vi "Process.vi"(8 "error in":errorcluster, 11 "XYStage":refnum<class "XYStage.lvclass">) -> (0 "error out":errorcluster, 3 "XYStage out":refnum<class "XYStage.lvclass">)   [LabVIEW 2017, in "XYStage.lvclass"]
doc: "---------------------------------------------------------------\nJKI State Machine Objects™\nhttp://jki.net/state-machine-objects/\nCopyright (C) 2005-2015, JKI <info@jki.net>\nALL RIGHTS RESERVEDJKI State Machine Objects (SMO) 1.0.0.5\nJKI - JKI\nCopyright (c) 2016, JKI"
uses:
  XYStage.lvclass
  D:/Program Files (x86)/National Instruments/LabVIEW 2017/vi.lib/JKI/JKI SMO/SMO/SMO.lvclass
  D:/upwork/Laser Measurement Tool/Laser/project/Subsystems/Device/Device.lvclass
  <vilib>/JKI/JKI SMO/SMO/Typedefs/Parent Call--Enum.ctl
  Typedefs/PublicEvents--XYStage.MoveCompleted.ctl
  Typedefs/Coordinates--Cluster.ctl
  Typedefs/Coordinates.Units--Cluster.ctl
  Typedefs/Coordinates.Counts--Cluster.ctl
  Typedefs/PublicEvents--XYStage.MoveStarted.ctl
  Device/Device.lvclass
  <vilib>/JKI/JKI SMO/SMO/SMO.lvclass
panel:
  # "XYStage\nProcess.vi"
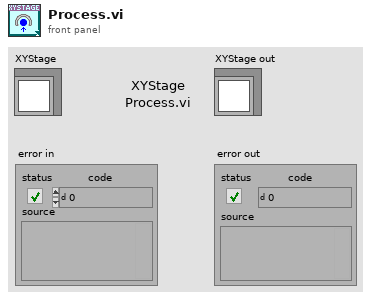
[diagram p1: front panel]
types:
  T1 = typedef "SMO.lvclass/Parent Call--Enum.ctl" = enum16{"Allows parent to run", "Does not request parent to run"}
  T2 = enum32{"invalid app kind", "Development System", "Run Time System", "Student Edition", "Embedded LabVIEW", "Evaluation", "Custom"}
  T3 = enum32{"Invalid", "Standard", "Closed", "Hidden", "Minimized", "Maximized"}
  T4 = typedef "XYStage.lvclass/PublicEvents--XYStage.MoveCompleted.ctl" = cluster{"Result":bool, "Coordinates":T5}
  T5 = typedef "XYStage.lvclass/Coordinates--Cluster.ctl" = cluster{"Units":T6, "Counts":T7}
  T6 = typedef "XYStage.lvclass/Coordinates.Units--Cluster.ctl" = cluster{"X":dbl, "Y":dbl}
  T7 = typedef "XYStage.lvclass/Coordinates.Counts--Cluster.ctl" = cluster{"X":i32, "Y":i32}
  T8 = typedef "Device.lvclass/PublicEvents--Device.Initialized.ctl" = bool
  T9 = cluster{"Core":cluster{"Current VI Reference":refnum<vi>, "Close Panel on Exit?":bool, "error":errorcluster}, "Self Reference":refnum<class "XYStage.lvclass">, "Initialized":bool, "Wait Timeout, ms":i32, "Target":T5, "Current":T5}
  T10 = cluster{"Current VI Reference":refnum<vi>, "Close Panel on Exit?":bool, "error":errorcluster}
  T11 = typedef "SMO.lvclass/Protected Events.ctl" = cluster{"StopProcesses":refnum<user-event>, "AbortProcesses":refnum<user-event>, "Config Changed":refnum<user-event>, "Dependency":refnum<user-event>}
  T12 = cluster{"Event Registration Refnum":refnum<event-registration>, "XYStage Protected Events":refnum<event-registration>, "Device Public Events":refnum<event-registration>, "XYStage Private Events":refnum<event-registration>}
  T13 = typedef "XYStage.lvclass/PublicEvents--XYStage.MoveStarted.ctl" = cluster{"Target":T5}
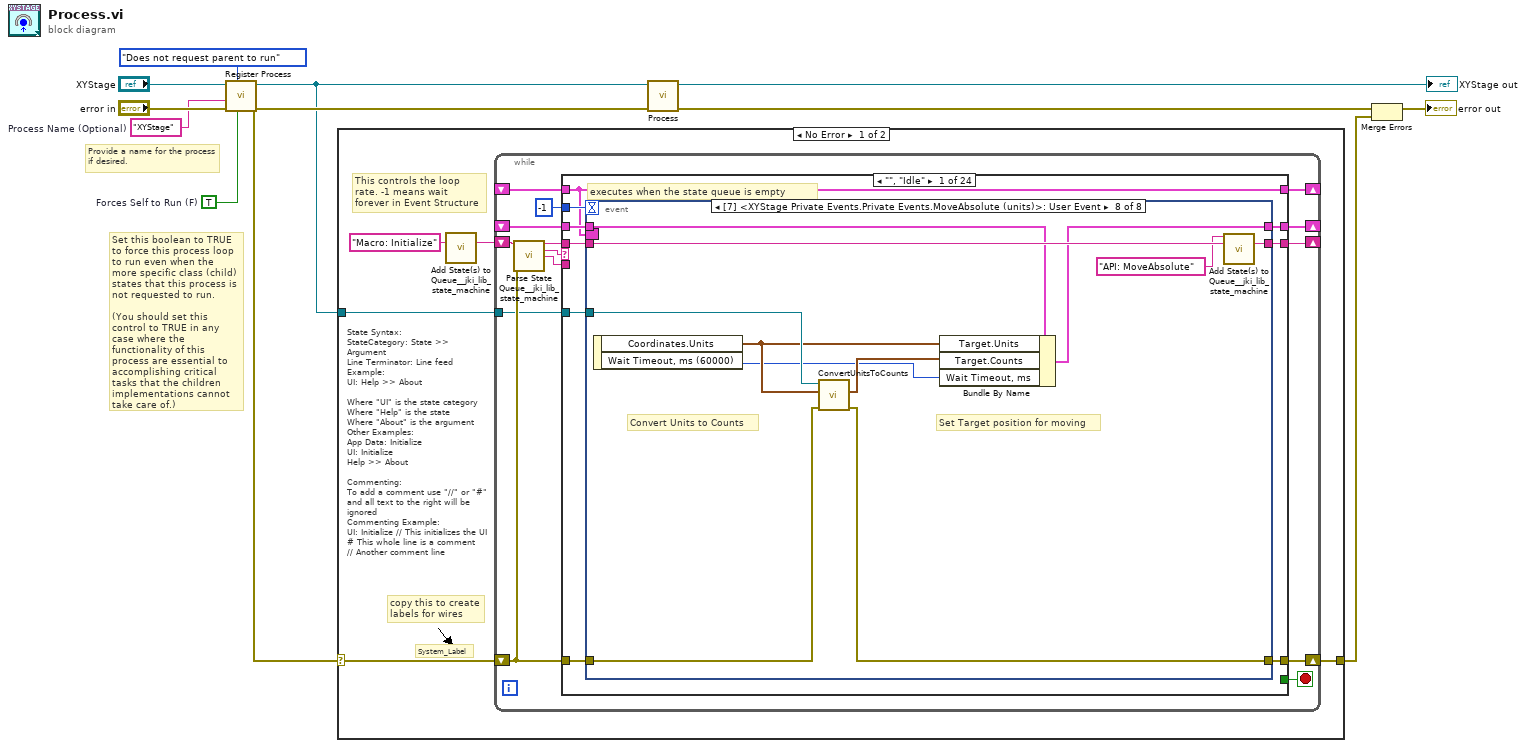
[diagram p0: block diagram]
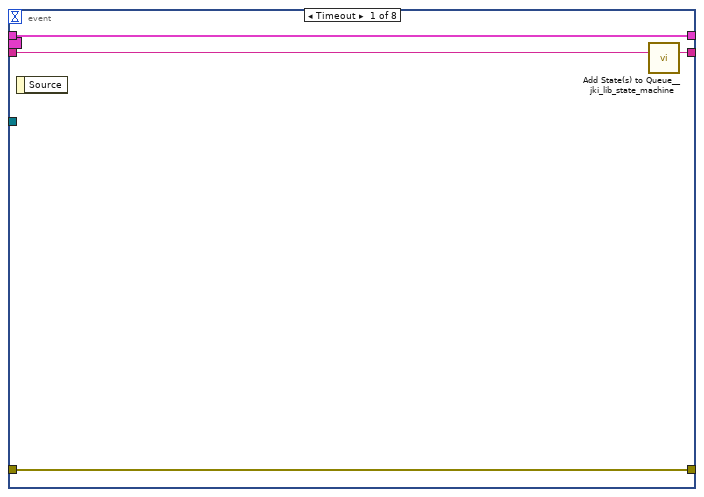
[diagram p2: hidden frame]
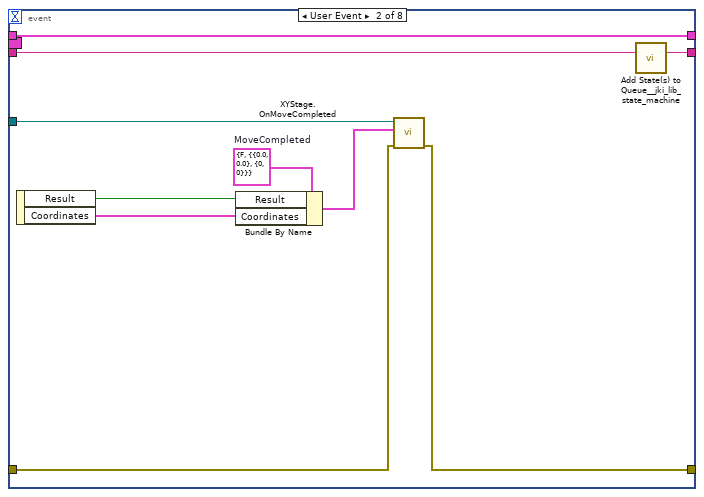
[diagram p3: hidden frame]
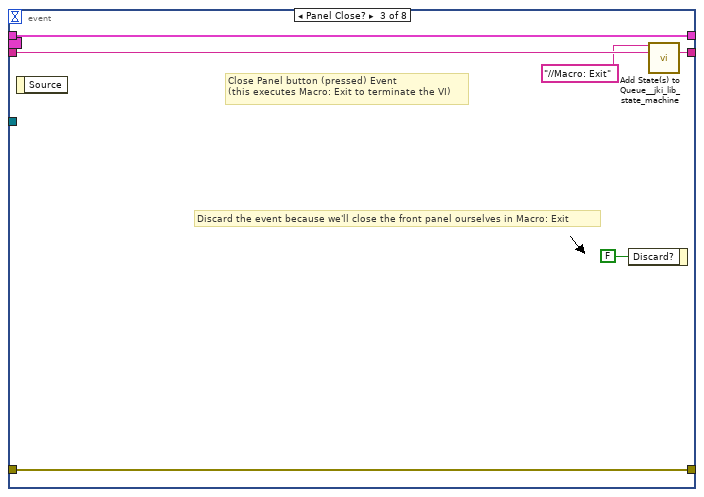
[diagram p4: hidden frame]
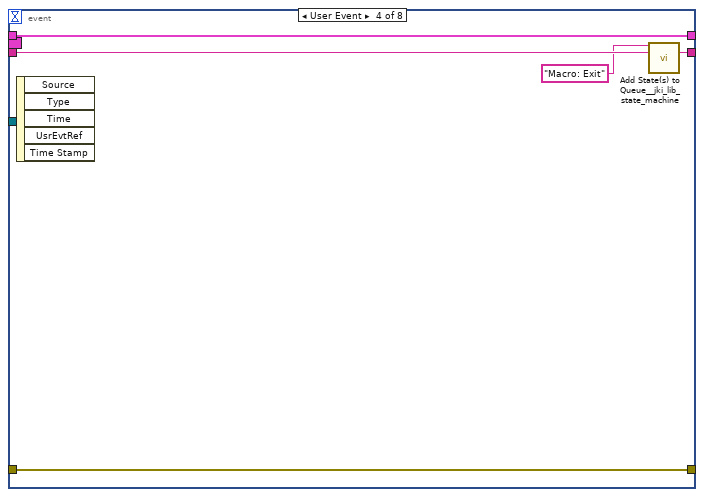
[diagram p5: hidden frame]
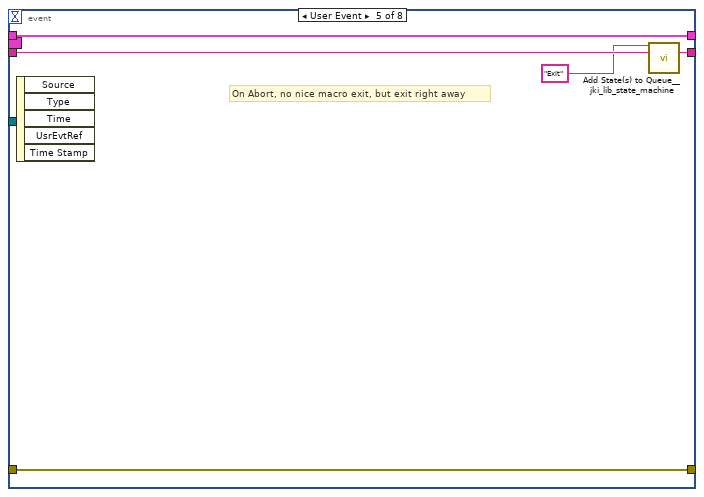
[diagram p6: hidden frame]
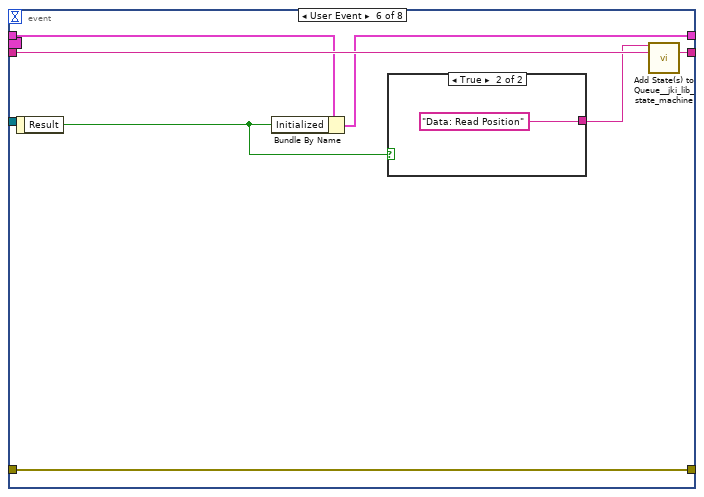
[diagram p7: hidden frame]
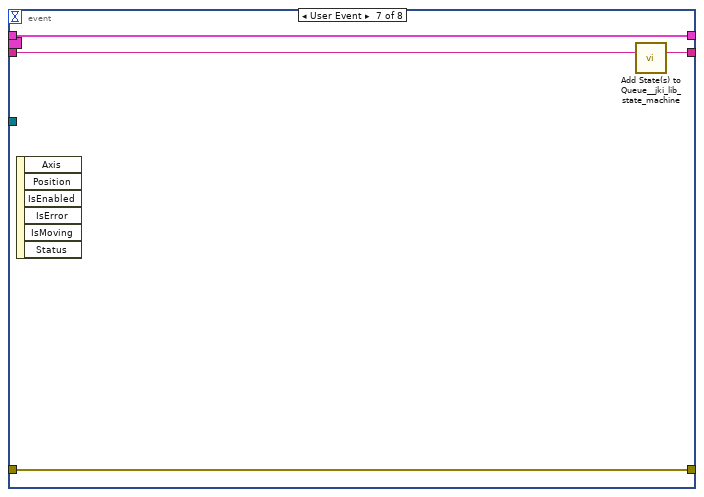
[diagram p9: hidden frame]
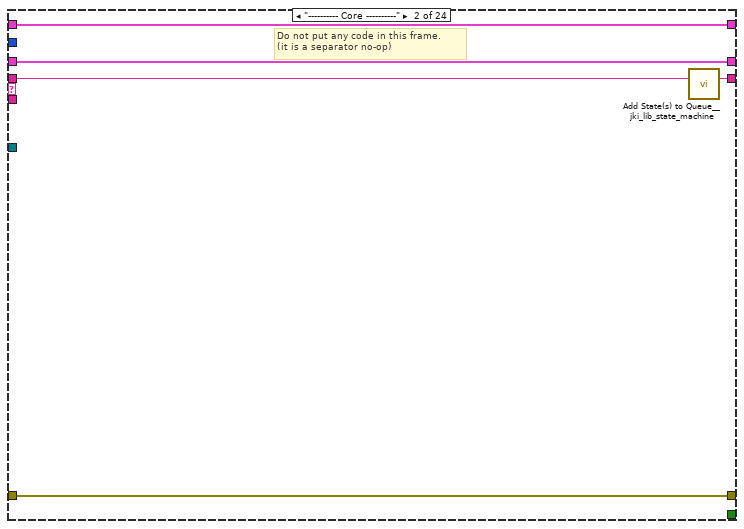
[diagram p10: hidden frame]
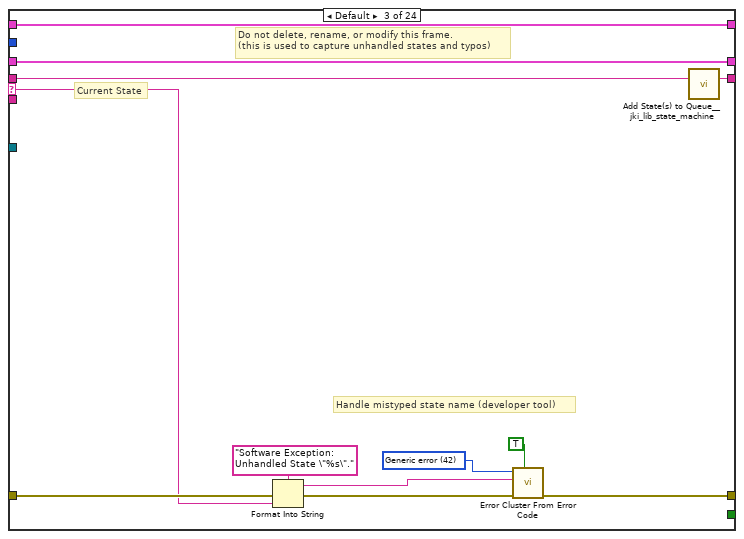
[diagram p11: hidden frame]
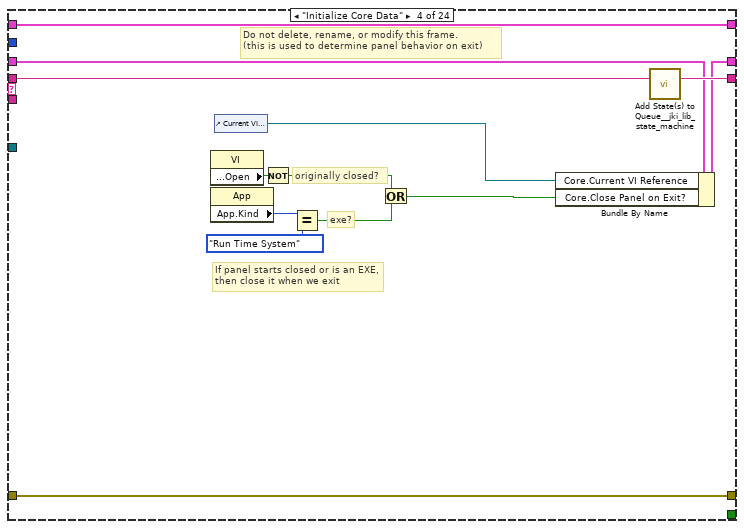
[diagram p12: hidden frame]
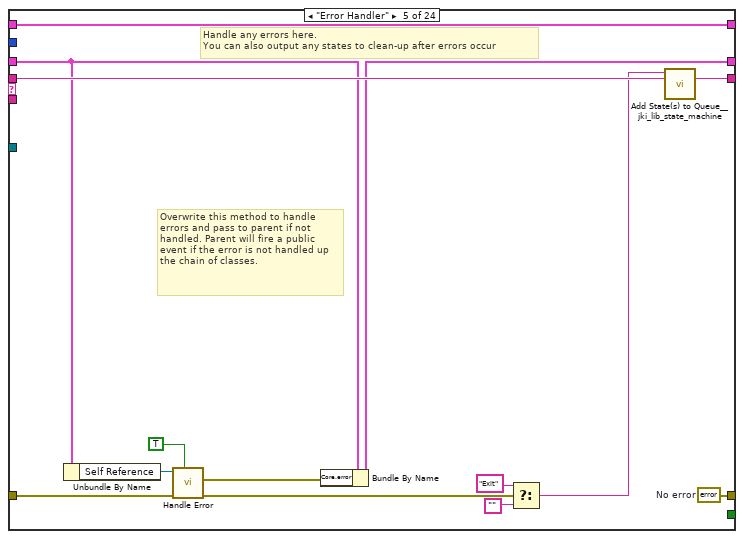
[diagram p13: hidden frame]
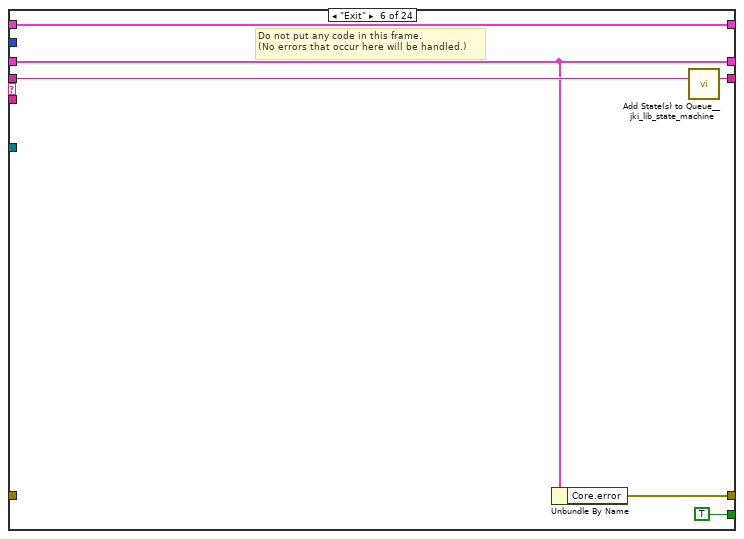
[diagram p14: hidden frame]
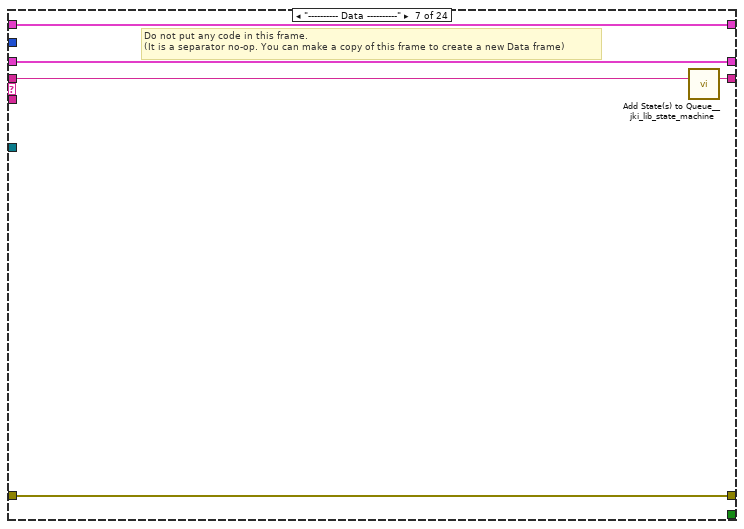
[diagram p15: hidden frame]
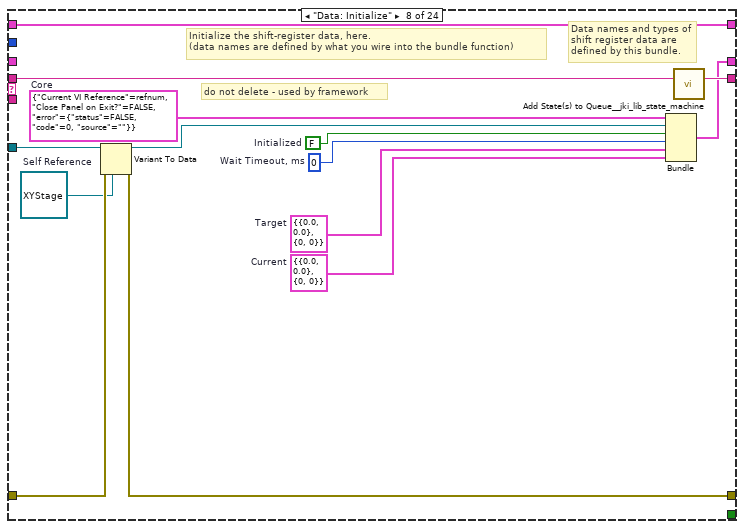
[diagram p16: hidden frame]
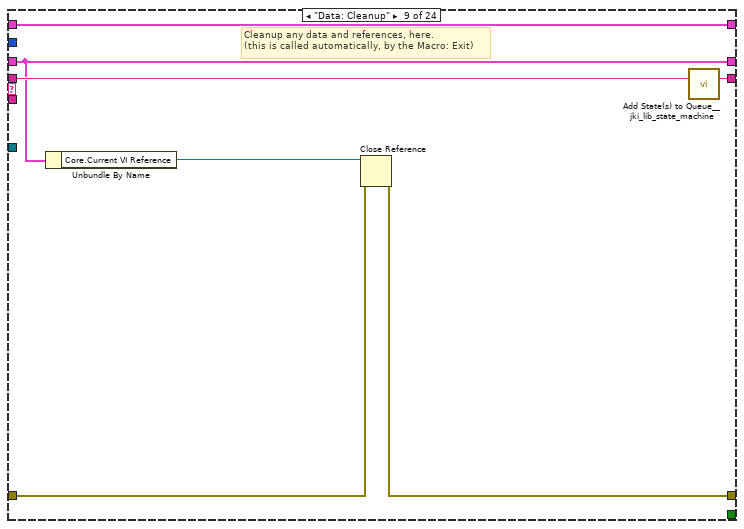
[diagram p17: hidden frame]
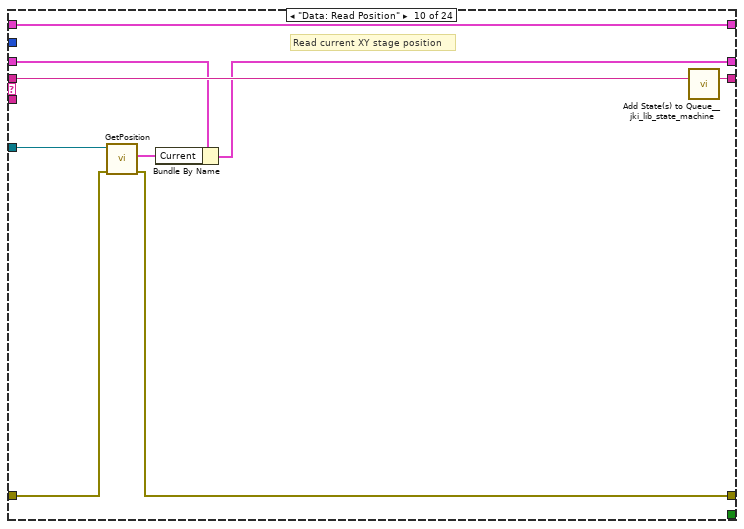
[diagram p18: hidden frame]
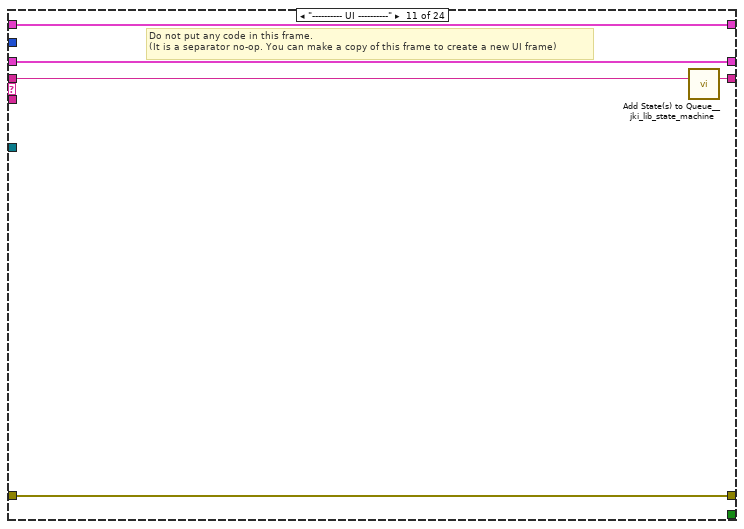
[diagram p19: hidden frame]
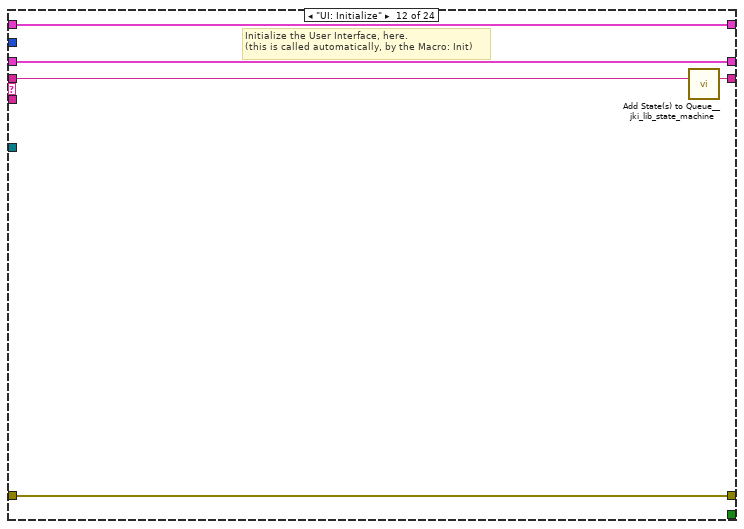
[diagram p20: hidden frame]
diagram:
  w2 = TRUE  # Forces Self to Run (F)
  w1 = "XYStage"  # Process Name (Optional)
  # "Provide a name for the process\nif desired."
  # "Set this boolean to TRUE to force this process loop to run even when the more specific class (child) states that this process is not requested to run.\n\n(You should set this control to TRUE in any case where the functionality of this process are essential to accomplishing critical tasks that the children implementations cannot take care of.)"
  n1 = call <vilib>:"Register Process.vi"("Forces Self to Run (F)"=w2, "Parent Call"=Parent_Call--Enum."Does not request parent to run", "error in (no error)"="error in", "Process Name (optional)"=w1, "SMO"="XYStage") -> ("error out"=w8:errorcluster, "SMO out"=w7:refnum<class "XYStage.lvclass">)  [unwired: 5 in]
  n2 = case shown="No Error" w8 {
    selector: w8 -> [w13 w332]
    tunnel: w7 -> [w14 _]
    tunnel: [w12 w332] -> w4
    frame No Error {
      # "State Syntax:\nStateCategory: State >> Argument\nLine Terminator: Line feed\nExample:\nUI: Help >> About\n\nWhere \"UI\" is the state category\nWhere \"Help\" is the state\nWhere \"About\" is the argument\nOther Examples:\nApp Data: Initialize\nUI: Initialize\nHelp >> About\n\nCommenting:\nTo add a comment use \"//\" or \"#\" and all text to the right will be ignored\nCommenting Example:\nUI: Initialize // This initializes the UI\n# This whole line is a comment\n// Another comment line"
      # "copy this to create labels for wires"
      # "This controls the loop rate. -1 means wait forever in Event Structure"
      # "System_Label"
      n3 = call <vilib>:"Add State(s) to Queue__jki_lib_state_machine.vi"("State(s) in (\"\")"="Macro: Initialize") -> ("States Out"=w16:string)  [unwired: 14 in]
      n4 = while {
        shift-right: [w23] -> _
        shift-left: _ -> [w22]
        shift-right: [w26] -> w12
        shift-left: w13 -> [w20]
        shift-right: [w25] -> _
        shift-left: w16 -> [w27]
        tunnel: w14 -> [w19]
        shift-right: [w18] -> _
        shift-left: _ -> [w17]
        stop <- w24 stop-if-true
        n5 = call <vilib>:"Parse State Queue__jki_lib_state_machine.vi"("State Queue"=w27, "Error In (no error)"=w20) -> ("Remaining States"=w29:string, "Current State"=w30:string, "Arguments"=w28:string)  [unwired: 11 in]
        n6 = case shown="\"\", \"Idle\"" w30 {
          selector: w30 -> [_ _ w99 _ _ _ _ _ _ _ _ _ _ _ _ _ _ _ _ _ _ _ _ _]
          tunnel: w29 -> [w39 w97 w103 w122 w136 w142 w147 w161 w168 w177 w182 w187 w194 w210 w242 w251 w265 w270 w281 w286 w306 w312 w317 w331]
          tunnel: w28 -> [_ _ _ _ _ _ _ _ _ _ _ _ w188 w204 _ _ _ _ _ _ _ _ _ _]
          tunnel: w22 -> [w37 w94 w101 w113 w125 w138 w144 _ w163 w172 w179 w185 w192 w206 w239 w247 w256 w267 w278 w283 w304 w310 w315 w322]
          tunnel: [w36 w95 w105 w119 w127 w137 w145 w157 w164 w170 w180 w184 w189 w207 w240 w249 w263 w268 w272 w284 w298 w308 w313 w323] -> w26
          tunnel: w20 -> [w35 w95 w104 w119 w132 _ w145 w158 w165 w173 w180 w184 w190 w208 w240 w249 w263 w268 w273 w284 w301 w308 w313 w326]
          tunnel: [w38 w96 w102 w121 w135 w141 w146 w160 w167 w176 w181 w186 w193 w209 w241 w250 w264 w269 w280 w285 w305 w311 w316 w330] -> w25
          tunnel: [_ _ _ _ _ TRUE _ _ _ _ _ _ _ _ _ _ _ _ _ _ _ _ _ _] -> w24
          tunnel: [w34 w94 w101 w120 w124 w138 w144 w159 w163 w169 w179 w185 w192 w206 w239 w247 w256 w267 w278 w283 w304 w310 w315 w322] -> w23
          tunnel: -1 ("Timeout") -> [w33 _ _ _ _ _ _ _ _ _ _ _ _ _ _ _ _ _ _ _ _ _ _ _]
          tunnel: w19 -> [w31 _ _ _ _ _ _ w155 _ w174 _ _ _ _ _ _ _ _ _ _ _ _ _ w321]
          tunnel: [w32 w93 w98 w110 w134 w139 w143 w153 w162 w175 w178 w183 w191 w203 w238 w248 w257 w266 w279 w282 w295 w309 w314 w329] -> w18
          tunnel: w17 -> [w32 w93 w98 w110 w134 w139 w143 w153 w162 w175 w178 w183 w191 w203 w238 w248 w257 w266 w279 w282 _ w309 w314 w329]
          frame "", "Idle" {
            # "executes when the state queue is empty"
            n7 = event shown="[7] <XYStage Private Events.Private Events.MoveAbsolute (units)>: User Event" {
              selector: w32 -> [_ _ _ _ _ _ _ _]
              dyn-events: _ -> [_ _ _ _ _ _ _ _]
              timeout: w33 -> [_ _ _ _ _ _ _ _]
              tunnel: w39 -> [w43 w44 w59 w64 w69 w76 w79 w91]
              tunnel: [w42 w45 w58 w63 w68 w75 w80 w92] -> w38
              tunnel: w37 -> [w40 w46 w56 w61 w66 w73 w81 w89]
              tunnel: [w41 w47 w57 w62 w67 w74 w78 w84] -> w36
              tunnel: w35 -> [w41 w48 w57 w62 w67 w74 w78 w85]
              tunnel: [w40 w46 w56 w61 w66 w72 w81 w88] -> w34
              tunnel: w31 -> [_ w51 _ _ _ _ _ w87]
              event Timeout {
                n8 = event-data() -> ()  [unwired: 1 in, 1 out]
                n9 = call <vilib>:"Add State(s) to Queue__jki_lib_state_machine.vi"("State(s) in (\"\")"=w43) -> ("States Out"=w42:string)  [unwired: 14 in]
              }
              event User Event {
                w52 = T4 {"Result"=FALSE, "Coordinates"={"Units"={"X"=0.0, "Y"=0.0}, "Counts"={"X"=0, "Y"=0}}}  # MoveCompleted
                n10 = event-data() -> ("Result"=w50:bool, "Coordinates"=w49:T5)  [unwired: 1 in]
                n11 = Bundle By Name(cluster=w52, "Result"=w50, "Coordinates"=w49) -> (w53:T4)
                n12 = call "XYStage.OnMoveCompleted.vi"("error in (no error)"=w48, "Move Completed"=w53, "XYStage"=w51) -> ("error out"=w47:errorcluster)  [unwired: 7 in, 1 out]
                n13 = call <vilib>:"Add State(s) to Queue__jki_lib_state_machine.vi"("State(s) in (\"\")"=w44) -> ("States Out"=w45:string)  [unwired: 14 in]
              }
              event Panel Close? {
                # "Discard the event because we'll close the front panel ourselves in Macro: Exit"
                # "Close Panel button (pressed) Event\n(this executes Macro: Exit to terminate the VI)"
                n14 = event-data() -> ()  [unwired: 1 in, 1 out]
                n15 = event-data("Discard?"=FALSE) -> ()  [unwired: 1 in, 1 out]
                n16 = call <vilib>:"Add State(s) to Queue__jki_lib_state_machine.vi"("State(s) in Front (\"\")"="//Macro: Exit", "State(s) in (\"\")"=w59) -> ("States Out"=w58:string)  [unwired: 13 in]
              }
              event User Event {
                n17 = event-data() -> ()  [unwired: 1 in, 5 out]
                n18 = call <vilib>:"Add State(s) to Queue__jki_lib_state_machine.vi"("State(s) in Front (\"\")"="Macro: Exit", "State(s) in (\"\")"=w64) -> ("States Out"=w63:string)  [unwired: 13 in]
              }
              event User Event {
                # "On Abort, no nice macro exit, but exit right away"
                n19 = event-data() -> ()  [unwired: 1 in, 5 out]
                n20 = call <vilib>:"Add State(s) to Queue__jki_lib_state_machine.vi"("State(s) in Front (\"\")"="Exit", "State(s) in (\"\")"=w69) -> ("States Out"=w68:string)  [unwired: 13 in]
              }
              event User Event {
                n21 = event-data() -> ("Result"=w71:T8)  [unwired: 1 in]
                n22 = Bundle By Name(cluster=w73, "Initialized"=w71) -> (w72:T9)
                n23 = case shown="True" w71 {
                  tunnel: [_ "Data: Read Position"] -> w70
                  frame False {
                  }
                  frame True {
                  }
                }
                n24 = call <vilib>:"Add State(s) to Queue__jki_lib_state_machine.vi"("State(s) in Front (\"\")"=w70, "State(s) in (\"\")"=w76) -> ("States Out"=w75:string)  [unwired: 13 in]
              }
              event User Event {
                n25 = event-data() -> ()  [unwired: 1 in, 6 out]
                n26 = call <vilib>:"Add State(s) to Queue__jki_lib_state_machine.vi"("State(s) in (\"\")"=w79) -> ("States Out"=w80:string)  [unwired: 14 in]
              }
              event User Event {
                # "Set Target position for moving"
                # "Convert Units to Counts"
                n27 = event-data() -> ("Coordinates.Units"=w83:T6, "Wait Timeout, ms (60000)"=w82:i32)  [unwired: 1 in]
                n28 = call "ConvertUnitsToCounts.vi"("error in (no error)"=w85, "Coordinates.Units"=w83, "XYStage in"=w87) -> ("error out"=w84:errorcluster, "Coordinates.Counts"=w86:T7)  [unwired: 6 in, 1 out]
                n29 = Bundle By Name(cluster=w89, "Target.Units"=w83, "Target.Counts"=w86, "Wait Timeout, ms"=w82) -> (w88:T9)
                n30 = call <vilib>:"Add State(s) to Queue__jki_lib_state_machine.vi"("State(s) in Front (\"\")"="API: MoveAbsolute", "State(s) in (\"\")"=w91) -> ("States Out"=w92:string)  [unwired: 13 in]
              }
            }
          }
          frame "---------- Core ----------" {
            # "Do not put any code in this frame.\n(it is a separator no-op)"
            n31 = call <vilib>:"Add State(s) to Queue__jki_lib_state_machine.vi"("State(s) in (\"\")"=w97) -> ("States Out"=w96:string)  [unwired: 14 in]
          }
          frame Default {
            w108 = 42 items=["No error", "Argument error", "Memory is full", "Out of zone", "End of file", "File already open", "Generic file I/O error", "File not found", "File permission error", "Disk is full", "Duplicate path", "Too many files open", "System feature not enabled", "Resource file not found", "Cannot add resource", "Resource not found", "Image not found", "Image memory error", "Pen does not exist", "Config type invalid", "Config token not found", "Config parse error", "Config memory error", "Bad external code format", "Bad external code offset", "External code not present", "Null window", "Destroy window error", "Null menu", "Print aborted", "Bad print record", "Print driver error", "Windows error during printing", "Memory error during printing", "Print dialog error", "Generic print error", "Invalid device refnum", "Device not found", "Device parameter error", "Device unit error", "Cannot open device", "Device call aborted", "Generic error", "Cancelled by user", "Object ID too low", "Object ID too high", "Object not in heap", "Unknown heap", "Unknown object (invalid DefProc)", "Unknown object (DefProc not in table)", "Message out of range", "Invalid (null) method", "Unknown message", "Manager call not supported", "Bad address", "Network operation in progress", "Network operation timed out", "Connection is busy", "Network attribute not supported", "Network error", "Address in use", "System out of memory", "Connection aborted", "Connection refused", "Not connected", "Already connected", "Connection closed", "Initialization error (interapplication manager)", "Bad occurrence", "Wait on unbound occurrence handler", "Occurrence queue overflow", "Datalog type conflict", "Unused", "Unrecognized type (interapplication manager)", "Memory corrupt", "Failed to make temporary DLL", "Old CIN version", "Drag socket not found", "Failed to load drop-object", "Failed to register OLE object", "Failed to release OLE object", "Format specifier type mismatch", "Unknown format specifier", "Too few format specifiers", "Too many format specifiers", "Scan failed", "Newer CIN version", "Error converting to variant", "Runtime menu error", "Password tampered", "Variant attribute not found", "Incompatible variant data type", "Event data is not available", "Event Store is not present", "Occurrence is not found", "Event Queue is not created", "Event info is not available", "Refnum passed is NULL", "Error retrieving Class GUID", "Error retrieving CoClass GUID", "Error retrieving TypeLib GUID.", "Bad built application magic bytes.", "Specific driver is different from the specific driver associated with the Logical Name.", "There is no session opened to the class driver.", "Max Error", "MAX - Error with config objects", "MAX - Error loading configuration", "MAX - Group not supported"]
            # "Current State"
            # "Do not delete, rename, or modify this frame.\n(this is used to capture unhandled states and typos)"
            # "Handle mistyped state name (developer tool)"
            n32 = Format Into String(format string="Software Exception: Unhandled State \"%s\"." ("message"), error in=w104, w99) -> (resulting string=w107:string, error out=w106:errorcluster)  [unwired: 1 in]
            n33 = call <vilib>:"Error Cluster From Error Code.vi"("show call chain? (False)"=TRUE, "error in (no error)"=w106, "error message (\"\")"=w107, "error code (0)"=w108) -> ("error out"=w105:errorcluster)  [unwired: 5 in]
            n34 = call <vilib>:"Add State(s) to Queue__jki_lib_state_machine.vi"("State(s) in (\"\")"=w103) -> ("States Out"=w102:string)  [unwired: 14 in]
          }
          frame "Initialize Core Data" {
            # "Do not delete, rename, or modify this frame.\n(this is used to determine panel behavior on exit)"
            # "originally closed?"
            # "exe?"
            # "If panel starts closed or is an EXE, then close it when we exit"
            n35 = property class="VI"() -> ("Front Panel.Open"=w118:bool)  [unwired: 2 in, 2 out]
            n36 = property class="App"() -> ("App.Kind"=w117:T2)  [unwired: 2 in, 2 out]
            n37 = control-ref of="Current VI Reference"() -> (w111:refnum<vi>)
            n38 = Not(x=w118) -> (.not. x?=w115:bool)
            n39 = Equal?(x=w117, y=T2."Run Time System" ("Application:Kind")) -> (x = y?=w114:bool)
            n40 = Or(x=w115, y=w114) -> (x .or. y?=w112:bool)
            n41 = Bundle By Name(cluster=w113, "Core.Current VI Reference"=w111, "Core.Close Panel on Exit?"=w112) -> (w120:T9)
            n42 = call <vilib>:"Add State(s) to Queue__jki_lib_state_machine.vi"("State(s) in (\"\")"=w122) -> ("States Out"=w121:string)  [unwired: 14 in]
          }
          frame "Error Handler" {
            w127 = errorcluster {"status"=FALSE, "code"=0, "source"=""}  # No error
            # "Overwrite this method to handle errors and pass to parent if not handled. Parent will fire a public event if the error is not handled up the chain of classes."
            # "Handle any errors here.\nYou can also output any states to clean-up after errors occur"
            n43 = Unbundle By Name(w125) -> ("Self Reference"=w133:refnum<class "XYStage.lvclass">)
            n44 = call-dynamic "Handle Error.vi"("Stop on Unhandled Error (T)"=TRUE, "error in"=w132, "SMO"=w133) -> ("handling error"=w128:errorcluster, "Unhandled error"=w126:errorcluster)  [unwired: 6 in, 1 out]
            n45 = Bundle By Name(cluster=w125, "Core.error"=w126) -> (w124:T9)
            n46 = Select(t="Exit", s=w128, f="") -> (s? t:f=w129:string)
            n47 = call <vilib>:"Add State(s) to Queue__jki_lib_state_machine.vi"("State(s) in Front (\"\")"=w129, "State(s) in (\"\")"=w136) -> ("States Out"=w135:string)  [unwired: 13 in]
          }
          frame "Exit" {
            # "Do not put any code in this frame.\n(No errors that occur here will be handled.)"
            n48 = Unbundle By Name(w138) -> ("Core.error"=w137:errorcluster)
            n49 = call <vilib>:"Add State(s) to Queue__jki_lib_state_machine.vi"("State(s) in (\"\")"=w142) -> ("States Out"=w141:string)  [unwired: 14 in]
          }
          frame "---------- Data ----------" {
            # "Do not put any code in this frame.\n(It is a separator no-op. You can make a copy of this frame to create a new Data frame)"
            n50 = call <vilib>:"Add State(s) to Queue__jki_lib_state_machine.vi"("State(s) in (\"\")"=w147) -> ("States Out"=w146:string)  [unwired: 14 in]
          }
          frame "Data: Initialize" {
            w148 = 0  # Wait Timeout, ms
            w149 = FALSE  # Initialized
            w150 = T5 {"Units"={"X"=0.0, "Y"=0.0}, "Counts"={"X"=0, "Y"=0}}  # Current
            w151 = T5 {"Units"={"X"=0.0, "Y"=0.0}, "Counts"={"X"=0, "Y"=0}}  # Target
            w152 = T10 {"Current VI Reference"=refnum, "Close Panel on Exit?"=FALSE, "error"={"status"=FALSE, "code"=0, "source"=""}}  # Core
            w156 = refnum<class "XYStage.lvclass"> refnum  # Self Reference
            # "do not delete - used by framework"
            # "Data names and types of shift register data are defined by this bundle."
            # "Initialize the shift-register data, here.\n(data names are defined by what you wire into the bundle function)"
            n51 = Variant To Data(error in=w158, type=w156, Variant=w155) -> (data=w154:refnum<class "XYStage.lvclass">, error out=w157:errorcluster)
            n52 = Bundle("Core"=w152, "Self Reference"=w154, "Initialized"=w149, "Wait Timeout, ms"=w148, "Target"=w151, "Current"=w150) -> (w159:T9)  [unwired: 1 in]
            n53 = call <vilib>:"Add State(s) to Queue__jki_lib_state_machine.vi"("State(s) in (\"\")"=w161) -> ("States Out"=w160:string)  [unwired: 14 in]
          }
          frame "Data: Cleanup" {
            # "Cleanup any data and references, here.\n(this is called automatically, by the Macro: Exit)"
            n54 = Unbundle By Name(w163) -> ("Core.Current VI Reference"=w166:refnum<vi>)
            n55 = Close Reference(reference=w166, error in (no error)=w165) -> (error out=w164:errorcluster)
            n56 = call <vilib>:"Add State(s) to Queue__jki_lib_state_machine.vi"("State(s) in (\"\")"=w168) -> ("States Out"=w167:string)  [unwired: 14 in]
          }
          frame "Data: Read Position" {
            # "Read current XY stage position"
            n57 = call "GetPosition.vi"("error in (no error)"=w173, "XYStage in"=w174) -> ("error out"=w170:errorcluster, "Coordinates"=w171:T5)  [unwired: 7 in, 1 out]
            n58 = Bundle By Name(cluster=w172, "Current"=w171) -> (w169:T9)
            n59 = call <vilib>:"Add State(s) to Queue__jki_lib_state_machine.vi"("State(s) in (\"\")"=w177) -> ("States Out"=w176:string)  [unwired: 14 in]
          }
          frame "---------- UI ----------" {
            # "Do not put any code in this frame.\n(It is a separator no-op. You can make a copy of this frame to create a new UI frame)"
            n60 = call <vilib>:"Add State(s) to Queue__jki_lib_state_machine.vi"("State(s) in (\"\")"=w182) -> ("States Out"=w181:string)  [unwired: 14 in]
          }
          frame "UI: Initialize" {
            # "Initialize the User Interface, here.\n(this is called automatically, by the Macro: Init)"
            n61 = call <vilib>:"Add State(s) to Queue__jki_lib_state_machine.vi"("State(s) in (\"\")"=w187) -> ("States Out"=w186:string)  [unwired: 14 in]
          }
          frame "UI: Cursor Set" {
            # "Argument"
            # "Initialize the User Interface, here.\n(this is called automatically, by the Macro: Init)"
            n62 = disable-structure shown="Default" {
              disable-tunnel: w190 -> [w195 w198]
              disable-tunnel: [w195 w197] -> w189
              disable-tunnel: w188 -> [_ w196]
              frame condition #0 {
              }
              frame condition #1 (active) {
                n63 = case shown="\"Idle\", Default" w196 {
                  tunnel: w198 -> [w200 w202]
                  tunnel: [w199 w201] -> w197
                  frame "Idle", Default {
                    n64 = call <vilib>:"Unset Busy.vi"("error in (no error)"=w200) -> ("error out"=w199:errorcluster)  [unwired: 10 in]
                  }
                  frame "Busy" {
                    n65 = call <vilib>:"Set Busy.vi"("error in (no error)"=w202) -> ("error out"=w201:errorcluster)  [unwired: 9 in, 1 out]
                  }
                }
              }
            }
            n66 = call <vilib>:"Add State(s) to Queue__jki_lib_state_machine.vi"("State(s) in (\"\")"=w194) -> ("States Out"=w193:string)  [unwired: 14 in]
          }
          frame "UI: Front Panel State" {
            # "Argument"
            # "Set Front Panel Open or Closed\n(Usage: \"UI: Front Panel State >> Open|Close\")"
            n67 = Unbundle By Name(w206) -> ("Core.Current VI Reference"=w205:refnum<vi>)
            n68 = disable-structure shown="Default" {
              disable-tunnel: w208 -> [w214 w237]
              disable-tunnel: [w213 w237] -> w207
              disable-tunnel: w205 -> [w212 _]
              disable-tunnel: w204 -> [w211 _]
              frame condition #0 (active) {
                n69 = case shown="\"Close\"" w211 {
                  tunnel: w214 -> [w218 w231]
                  tunnel: [w220 w232] -> w213
                  tunnel: w212 -> [w219 w229]
                  frame "Open", Default {
                    n70 = property class="VI"(reference=w219, error in=w218) -> (reference out=w216:refnum<vi>, error out=w217:errorcluster, "FP.State"=w215:T3)
                    n71 = case shown="\"Closed\"" w215 {
                      tunnel: [w223 w226] -> w220
                      tunnel: w217 -> [w222 w226]
                      tunnel: w216 -> [w221 _]
                      frame "Closed" {
                        n72 = invoke class="VI" method="FP.Open"(reference=w221, error in=w222, "Activate"=TRUE, "State"=T3."Standard") -> (error out=w223:errorcluster)  [unwired: 1 in, 4 out]
                      }
                      frame Default {
                      }
                    }
                  }
                  frame "Close" {
                    n73 = property class="VI"(reference=w229, error in=w231) -> (reference out=w228:refnum<vi>, error out=w230:errorcluster, "FP.State"=w227:T3)
                    n74 = case shown="Default" w227 {
                      tunnel: [w233 w236] -> w232
                      tunnel: w230 -> [w233 w235]
                      tunnel: w228 -> [_ w234]
                      frame "Invalid", "Closed" {
                      }
                      frame Default {
                        n75 = invoke class="VI" method="FP.Close"(reference=w234, error in=w235) -> (error out=w236:errorcluster)  [unwired: 1 in, 2 out]
                      }
                    }
                  }
                }
              }
              frame condition #1 {
              }
            }
            n76 = call <vilib>:"Add State(s) to Queue__jki_lib_state_machine.vi"("State(s) in (\"\")"=w210) -> ("States Out"=w209:string)  [unwired: 14 in]
          }
          frame "---------- Macro ----------" {
            # "Do not put any code in this frame.\n(It is a separator no-op. You can make a copy of this frame to create a new Macro frame)"
            n77 = call <vilib>:"Add State(s) to Queue__jki_lib_state_machine.vi"("State(s) in (\"\")"=w242) -> ("States Out"=w241:string)  [unwired: 14 in]
          }
          frame "Macro: Initialize" {
            w245 = "UI: Initialize\n//UI: Front Panel State >> Open"  # UI: Initialize //UI: Front Panel State >> Open
            # "Initialization Macro\n(This is called once, when the VI starts)"
            n78 = call <vilib>:"Add State(s) to Queue__jki_lib_state_machine.vi"("State(s) in Front (\"\")"="Data: Initialize\nInitialize Core Data\nEvents: Register", "State(s) in (\"\")"="Process: Sync", "State(s) at Back (\"\")"=w245) -> ("States Out"=w244:string)  [unwired: 12 in]
            n79 = call <vilib>:"Add State(s) to Queue__jki_lib_state_machine.vi"("State(s) in Front (\"\")"=w244, "State(s) in (\"\")"=w251) -> ("States Out"=w250:string)  [unwired: 13 in]
          }
          frame "Macro: Exit" {
            # "Exit Macro\n(This is called once, when the VI exits)"
            n80 = Unbundle By Name(w256) -> ("Core.Close Panel on Exit?"=w262:bool)
            n81 = Select(t="UI: Front Panel State >> Close", s=w262, f="") -> (s? t:f=w259:string)
            n82 = call <vilib>:"Add State(s) to Queue__jki_lib_state_machine.vi"("State(s) in Front (\"\")"="Data: Cleanup\nEvents: Unregister", "State(s) in (\"\")"="Process: Sync", "State(s) at Back (\"\")"="Exit") -> ("States Out"=w253:string)  [unwired: 12 in]
            n83 = call <vilib>:"Add State(s) to Queue__jki_lib_state_machine.vi"("State(s) in (\"\")"=w259, "State(s) at Back (\"\")"=w253) -> ("States Out"=w258:string)  [unwired: 13 in]
            n84 = call <vilib>:"Add State(s) to Queue__jki_lib_state_machine.vi"("State(s) in Front (\"\")"=w258, "State(s) in (\"\")"=w265) -> ("States Out"=w264:string)  [unwired: 13 in]
          }
          frame "---------- Process ----------" {
            # "Template Separator\n(You can make a copy of, or modify, this frame)"
            n85 = call <vilib>:"Add State(s) to Queue__jki_lib_state_machine.vi"("State(s) in (\"\")"=w270) -> ("States Out"=w269:string)  [unwired: 14 in]
          }
          frame "Process: Sync" {
            n86 = Unbundle By Name(w278) -> ("Self Reference"=w274:refnum<class "XYStage.lvclass">)
            n87 = call <vilib>:"WaitOnProcessSync.vi"("error in (no error)"=w273, "SMO"=w274) -> ("error out"=w272:errorcluster, "Don't run?"=w277:bool)  [unwired: 7 in, 1 out]
            n88 = Select(t="Data: Cleanup\nEvents: Unregister\nExit", s=w277, f="") -> (s? t:f=w271:string)
            n89 = call <vilib>:"Add State(s) to Queue__jki_lib_state_machine.vi"("State(s) in Front (\"\")"=w271, "State(s) in (\"\")"=w281) -> ("States Out"=w280:string)  [unwired: 13 in]
          }
          frame "---------- Events ----------" {
            # "Template Separator\n(You can make a copy of, or modify, this frame)"
            n90 = call <vilib>:"Add State(s) to Queue__jki_lib_state_machine.vi"("State(s) in (\"\")"=w286) -> ("States Out"=w285:string)  [unwired: 14 in]
          }
          frame "Events: Register" {
            # "XYStage Private Events"
            # "Device Public Events"
            # "XYStage Protected Events"
            # "Base Class Protected Events"
            n91 = Unbundle By Name(w304) -> ("Self Reference"=w302:refnum<class "XYStage.lvclass">)
            n92 = call <vilib>:"GetProtectedEvents.vi"("SMO"=w302) -> ("error out"=w299:errorcluster, "SMO Protected Events"=w303:T11, "SMO out"=w290:refnum<class "XYStage.lvclass">)  [unwired: 8 in]
            n93 = call "XYStage.GetProtectedEventsRegistration.vi"("XYStage in"=w290) -> ("error out"=w288:errorcluster, "XYStage Protected Events"=w287:refnum<event-registration>, "XYStage out"=w289:refnum<class "XYStage.lvclass">)  [unwired: 8 in]
            n94 = call "Device.GetPublicEventsRegistration.vi"("Device in"=w289) -> ("error out"=w294:errorcluster, "Device Public Events"=w296:refnum<event-registration>, "Device out"=w293:refnum<class "XYStage.lvclass">)  [unwired: 8 in]
            n95 = call "XYStage.GetPrivateEventsRegistration.vi"("XYStage in"=w293) -> ("error out"=w291:errorcluster, "XYStage Private Events"=w292:refnum<event-registration>)  [unwired: 8 in, 1 out]
            n96 = register-events(w303) -> (reference out=w297:refnum<event-registration>, error out=w300:errorcluster)  [unwired: 2 in]
            n97 = Bundle("Event Registration Refnum"=w297, "XYStage Protected Events"=w287, "Device Public Events"=w296, "XYStage Private Events"=w292) -> (w295:T12)  [unwired: 1 in]
            n98 = Merge Errors(w291, w301, w294, w300, w288, w299) -> (w298:errorcluster)
            n99 = call <vilib>:"Add State(s) to Queue__jki_lib_state_machine.vi"("State(s) in (\"\")"=w306) -> ("States Out"=w305:string)  [unwired: 14 in]
          }
          frame "Events: Unregister" {
            n100 = Unregister For Events(event registration refnum=w309, error in=w308) -> (error out=w307:errorcluster)
            n101 = call <vilib>:"Clear Errors.vi"("error in (no error)"=w307) -> ()  [unwired: 5 in, 2 out]
            n102 = call <vilib>:"Add State(s) to Queue__jki_lib_state_machine.vi"("State(s) in (\"\")"=w312) -> ("States Out"=w311:string)  [unwired: 14 in]
          }
          frame "---------- API ----------" {
            n103 = call <vilib>:"Add State(s) to Queue__jki_lib_state_machine.vi"("State(s) in (\"\")"=w317) -> ("States Out"=w316:string)  [unwired: 14 in]
          }
          frame "API: MoveAbsolute" {
            w328 = T13 {"Target"={"Units"={"X"=0.0, "Y"=0.0}, "Counts"={"X"=0, "Y"=0}}}  # MoveStarted
            n104 = Unbundle By Name(w322) -> ("Target"=w320:T5, "Wait Timeout, ms"=w318:i32)
            n105 = Unbundle By Name(w320) -> ("Counts"=w319:T7)
            n106 = Bundle By Name(cluster=w328, "Target"=w320) -> (w327:T13)
            n107 = call "XYStage.OnMoveStarted.vi"("error in (no error)"=w326, "MoveStarted"=w327, "XYStage"=w321) -> ("error out"=w324:errorcluster, "XYStage out"=w325:refnum<class "XYStage.lvclass">)  [unwired: 7 in]
            n108 = call-dynamic "XYStage.MoveAbsolute (counts).vi"("Wait Timeout, ms (60000)"=w318, "error in (no error)"=w324, "Counts"=w319, "XYStage in"=w325) -> ("error out"=w323:errorcluster)  [unwired: 6 in, 1 out]
            n109 = call <vilib>:"Add State(s) to Queue__jki_lib_state_machine.vi"("State(s) in (\"\")"=w331) -> ("States Out"=w330:string)  [unwired: 14 in]
          }
        }
      }
    }
    frame Error {
    }
  }
  n110 = call-parent "Process.vi"("error in"=w8, "SMO"=w7) -> ("error out"=w5:errorcluster, "SMO out"=→"XYStage out":refnum<class "XYStage.lvclass">)  [unwired: 8 in]
  n111 = Merge Errors(w5, w4) -> (→"error out":errorcluster)
